vi "DegreesToRadians.vi"(1 "Degrees":dbl) -> (0 "Radians":dbl)   [LabVIEW 2016]
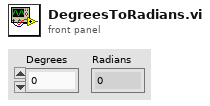
[diagram p1: front panel]
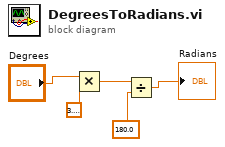
[diagram p0: block diagram]
diagram:
  n1 = Multiply(x="Degrees", y=3.141592653589793) -> (x*y=w2:dbl)
  n2 = Divide(x=w2, y=180.0) -> (x/y=→"Radians":dbl)
